vi "Reset All Output Modulo Counters.vi"(8 "error in (no error)":errorcluster) -> (0 "error out":errorcluster)   [LabVIEW 2009]
doc: "long ResetAllOutputModuloCounters(void);"
uses:
  DelayGenerator.dll
panel:
  # "NOTICE -- YOU MUST LEAVE THIS NOTICE IN PLACE.  PER THE TERMS OF THE LICENSE BELOW, YOU MAY SUBLICENSE THIS SOFTWARE \nIN ANY WAY THAT DOES NOT CONFLICT WITH THIS LICENSE.\n\n### BSD License (http://www.opensource.org/licenses/bsd-license.php) Begin ###\n \nCopyright (c) 2011, Applied Energetics, http://www.appliedenergetics.com,\n                               Richard Schwerdtfeger, <rschwerdtfeger@appliedenergetics.com>\n\nAll rights reserved.\n\nRedistribution and use in source and binary forms, with or without modification, are permitted provided that the \nfollowing conditions are met:\n\n    * Redistributions of source code must retain the above copyright notice, this list of conditions and the following disclaimer.\n    * Redistributions in binary form must reproduce the above copyright notice, this list of conditions and the following disclaimer \n       in the documentation and/or other materials provided with the distribution.\n    * Neither the name of Richard Schwerdtfeger, Applied Energetics, Inc., nor the names of its contributors may be used to \n       endorse or promote products derived from this software without specific prior written permission.\n\nTHIS SOFTWARE IS PROVIDED BY THE COPYRIGHT HOLDERS AND CONTRIBUTORS \"AS IS\" AND ANY EXPRESS OR IMPLIED WARRANTIES, \nINCLUDING, BUT NOT LIMITED TO, THE IMPLIED WARRANTIES OF MERCHANTABILITY AND FITNESS FOR A PARTICULAR PURPOSE ARE \nDISCLAIMED. IN NO EVENT SHALL THE COPYRIGHT OWNER OR CONTRIBUTORS BE LIABLE FOR ANY DIRECT, INDIRECT, INCIDENTAL,\n SPECIAL, EXEMPLARY, OR CONSEQUENTIAL DAMAGES (INCLUDING, BUT NOT LIMITED TO, PROCUREMENT OF SUBSTITUTE GOODS OR \nSERVICES; LOSS OF USE, DATA, OR PROFITS; OR BUSINESS INTERRUPTION) HOWEVER CAUSED AND ON ANY THEORY OF LIABILITY, \nWHETHER IN CONTRACT, STRICT LIABILITY, OR TORT (INCLUDING NEGLIGENCE OR OTHERWISE) ARISING IN ANY WAY OUT OF THE USE \nOF THIS SOFTWARE, EVEN IF ADVISED OF THE POSSIBILITY OF SUCH DAMAGE.\n\n### BSD License End ###"
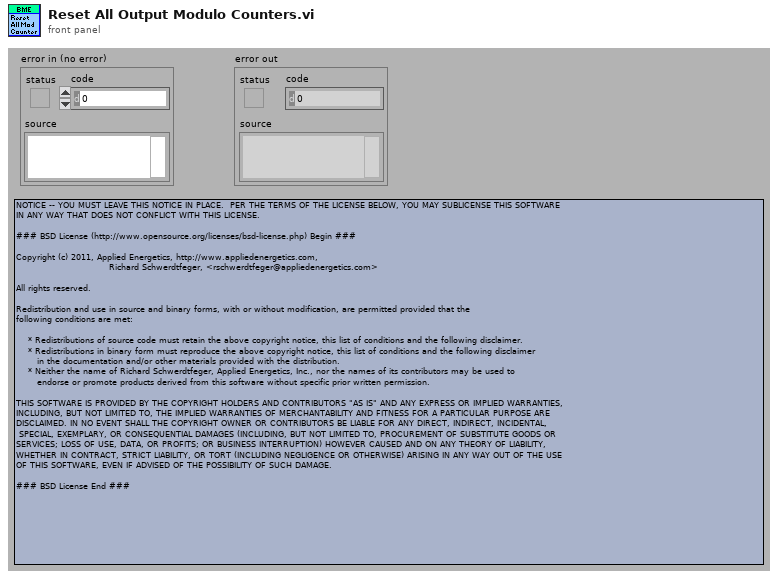
[diagram p1: front panel]
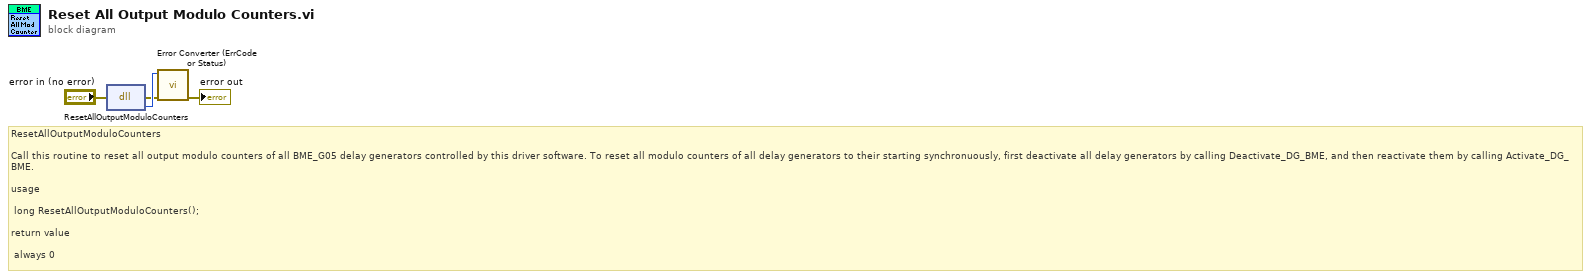
[diagram p0: block diagram]
diagram:
  # "ResetAllOutputModuloCounters\n\nCall this routine to reset all output modulo counters of all BME_G05 delay generators controlled by this driver software. To reset all modulo counters of all delay generators to their starting synchronuously, first deactivate all delay generators by calling Deactivate_DG_BME, and then reactivate them by calling Activate_DG_BME.\n\nusage\n\n\tlong ResetAllOutputModuloCounters();\n\nreturn value\n\n\talways 0"
  n1 = dll-call lib="C:/Dokumente und Einstellungen/A2.5/Desktop/BME_SW Stand 201203-26/LabView_SG08p/BME Delay Generator/DelayGenerator.*" fn="ResetAllOutputModuloCounters"(error in="error in (no error)") -> (error out=w2:errorcluster, w4:i32)  [unwired: 2 in, 1 out]
  n2 = call "Error Converter (ErrCode or Status).vi"("error in (no error)"=w2, "error code"=w4) -> ("error out"=→"error out":errorcluster)  [unwired: 9 out]
